vi "z chunk alloc result new error.vi"(8 "error in (no error)":errorcluster, 10 "alloc_error":u32(ring) items=["Z_ALLOC_ERROR_NEED_DEFRAGMENT", "Z_ALLOC_ERROR_OUT_OF_MEMORY", "Z_ALLOC_ERROR_OTHER"], 11 "this_":cluster{}) -> (0 "error out":errorcluster, 3 "this_ out":cluster{})   [LabVIEW 2021, in "zenohc.lvlib"]
doc: "void z_chunk_alloc_result_new_error(struct z_owned_chunk_alloc_result_t *this_,\n enum z_alloc_error_t alloc_error);"
uses:
  zenohc.lvlib
  zenohc.dll
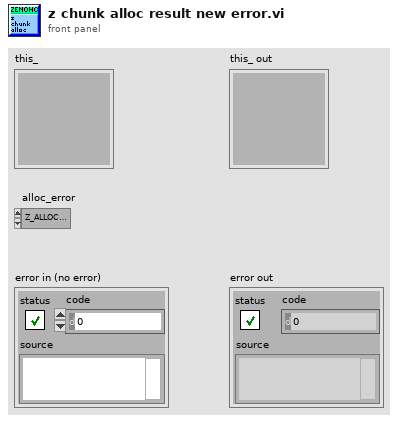
[diagram p1: front panel]
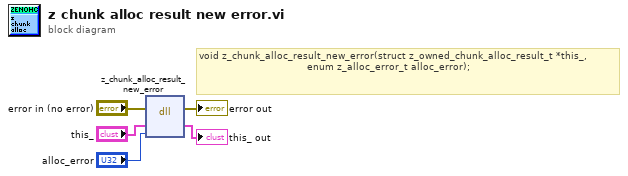
[diagram p0: block diagram]
diagram:
  # "void z_chunk_alloc_result_new_error(struct z_owned_chunk_alloc_result_t *this_,\n                                    enum z_alloc_error_t alloc_error);"
  n1 = dll-call lib="D:/dev/zenoh_labview/zenohc/zenohc.*" fn="z_chunk_alloc_result_new_error"(error in="error in (no error)", "this_"="this_", "alloc_error"="alloc_error") -> (error out=→"error out":errorcluster, "this_"=→"this_ out":cluster{})  [unwired: 4 in, 1 out]
